vi "analyse.vi"(11 "Refnum in":T1) -> (3 "Centroid":cluster{"X Centroid":sgl, "Y Centroid":sgl})   [LabVIEW 2011, in "MoveDataFile.lvclass"]
uses:
  MoveDataFile.lvclass
  <vilib>/vision/Image Controls.llb/IMAQ Image.ctl
  shared/CompressAndUpdate(Poly)/CompressAndUpdate(Numeric).vi
  <vilib>/vision/NI_Vision_Development_Module.lvlib
  <vilib>/Analysis/NI_AALBase.lvlib
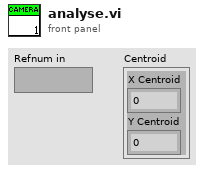
[diagram p1: front panel]
types:
  T1 = typedef "IMAQ Image.ctl" = refnum<image>
  T2 = typedef "Image Type" = u32
  T3 = cluster{"histogram":u32[], "Minimal Value":sgl, "Maximal Value":sgl, "Starting Value":sgl, "Interval Width":sgl, "Mean Value":sgl, "Standard  Variation":sgl, "Area (pixels)":i32}
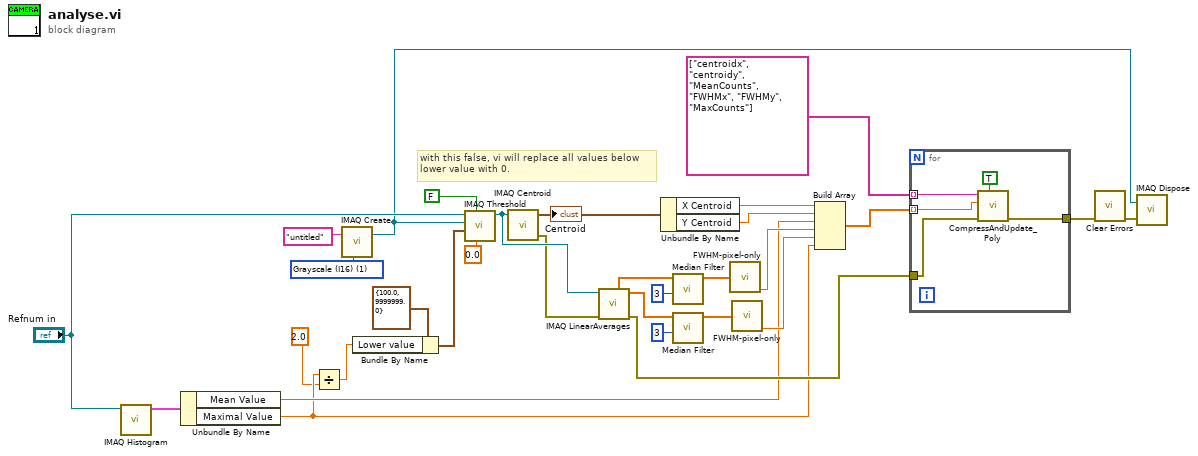
[diagram p0: block diagram]
diagram:
  w27 = T2 1 items=["Grayscale (U8)", "Grayscale (I16)", "Grayscale (SGL)", "Complex (CSG)", "RGB (U32)", "HSL (U32)", "RGB (U64)", "Grayscale (U16)"] ("Image Type")
  # "with this false, vi will replace all values below\nlower value with 0."
  n1 = call "IMAQ Histogram"("Image"="Refnum in") -> ("Histogram Report"=w7:T3)  [unwired: 9 in, 1 out]
  n2 = Unbundle By Name(w7) -> ("Mean Value"=w5:sgl, "Maximal Value"=w3:sgl)
  n3 = Divide(x=w3, y=sgl 2.0) -> (x/y=w1:sgl)
  n4 = call "IMAQ Create"("Image Name"="untitled", "Image Type"=w27) -> ("New Image"=w4:T1)  [unwired: 3 in, 1 out]
  n5 = Bundle By Name(cluster=cluster{"Lower value":sgl, "Upper value":sgl} {"Lower value"=100.0, "Upper value"=9999999.0} ("Range"), "Lower value"=w1) -> (w31:cluster{"Lower value":sgl, "Upper value":sgl})
  n6 = call "IMAQ Threshold"("Replace Value"=sgl 0.0, "Keep/Replace Value (Replace)"=FALSE, "Range"=w31, "Image Dst"=w4, "Image Src"="Refnum in") -> ("Image Dst Out"=w18:T1)  [unwired: 5 in, 1 out]
  n7 = call "IMAQ Centroid"("Image"=w18) -> ("error out"=w9:errorcluster, "Centroid"=w25:cluster{"X Centroid":sgl, "Y Centroid":sgl})  [unwired: 3 in]
  "Centroid" <- w25
  n8 = call "IMAQ LinearAverages"("error in (no error)"=w9, "Image Src"=w18) -> ("error out"=w8:errorcluster, "Y Axis Averages"=w17:sgl[], "X Axis Averages"=w13:sgl[])  [unwired: 2 in, 5 out]
  n9 = Unbundle By Name(w25) -> ("X Centroid"=w22:sgl, "Y Centroid"=w21:sgl)
  n10 = call <vilib>:"Median Filter.vi"("right rank"=3 ("left rank"), "X"=w13) -> ("Filtered X"=w12:dbl[])  [unwired: 8 in, 1 out]
  n11 = call <vilib>:"Median Filter.vi"("right rank"=3 ("left rank"), "X"=w17) -> ("Filtered X"=w15:dbl[])  [unwired: 8 in, 1 out]
  n12 = call "FWHM-pixel-only.vi"("lineout"=w12) -> ("FWHM (pix)"=w11:dbl)  [unwired: 2 in, 1 out]
  n13 = call "FWHM-pixel-only.vi"("lineout"=w15) -> ("FWHM (pix)"=w10:dbl)  [unwired: 2 in, 1 out]
  n14 = Build Array(w22, w21, w5, w11, w10, w3) -> (w23:dbl[])
  n15 = for {
    tunnel: string[] ["centroidx", "centroidy", "MeanCounts", "FWHMx", "FWHMy", "MaxCounts"] -> [w36] mode=indexing
    tunnel: w23 -> [w35] mode=indexing
    tunnel: w8 -> [w34]
    tunnel: [w33] -> w20
    n16 = call-poly "CompressAndUpdate_Poly.vi"("force CVT update (false)"=TRUE, "error in"=w34, "Numeric"=w35, "command or variable name"=w36) -> ("error out"=w33:errorcluster)  [unwired: 7 in]
  }
  n17 = call <vilib>:"Clear Errors.vi"("error in (no error)"=w20) -> ("error out"=w19:errorcluster)  [unwired: 6 in]
  n18 = call "IMAQ Dispose"("Image"=w4, "error in (no error)"=w19) -> ()  [unwired: 4 in, 1 out]
